vi "Check Valid Message.vi"(8 "error in (no error)":errorcluster, 10 "Message":string, 11 "Passive Hardware in":refnum<class "Passive Hardware.lvclass">) -> (0 "error out":errorcluster, 2 "Valid?":bool, 3 "Passive Hardware out":refnum<class "Passive Hardware.lvclass">)   [LabVIEW 2020, in "RxnRover.lvlib" / "Passive Hardware.lvclass"]
doc: "Checks if a message recieved from a Passive-Hardware instrument is valid by comparing it to a list of valid messages. \n\nRxnRover 2025"
uses:
  Passive Hardware.lvclass
  Passive Hardware.lvclass/Passive Hardware.ctl
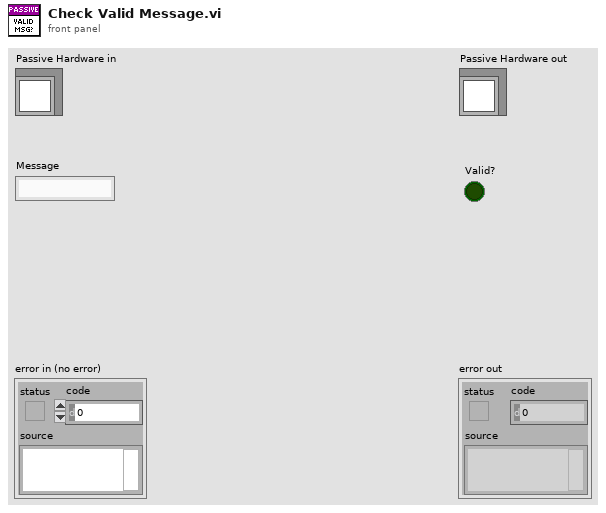
[diagram p1: front panel]
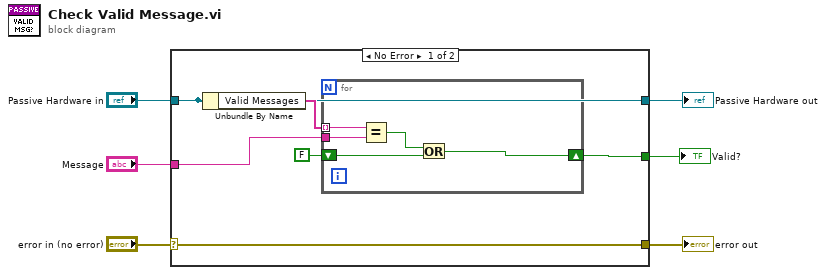
[diagram p0: block diagram]
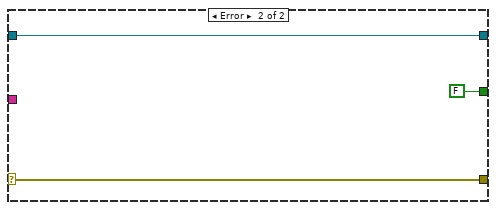
[diagram p2: hidden frame]
diagram:
  n1 = case shown="No Error" "error in (no error)" {
    selector: "error in (no error)" -> [w9 w19]
    tunnel: [w12 FALSE ("Valid?")] -> w2
    tunnel: "Passive Hardware in" -> [w8 w20]
    tunnel: "Message" -> [w11 _]
    tunnel: [w9 w19] -> w3
    tunnel: [w8 w20] -> w1
    frame No Error {
      n2 = Unbundle By Name(w8) -> ("Valid Messages"=w10:string[])
      n3 = for {
        tunnel: w10 -> [w16] mode=indexing
        tunnel: w11 -> [w17]
        shift-right: [w13] -> w12
        shift-left: FALSE -> [w14]
        n4 = Equal?(x=w16, y=w17) -> (x = y?=w15:bool)
        n5 = Or(x=w15, y=w14) -> (x .or. y?=w13:bool)
      }
    }
    frame Error {
    }
  }
  "error out" <- w3
  "Passive Hardware out" <- w1
  "Valid?" <- w2
